vi "Insert Channel Create Params.vi"(8 "error in":errorcluster, 11 "TDMS in":refnum<class "TDMS.lvclass">) -> (0 "error out":errorcluster, 3 "TDMS out":refnum<class "TDMS.lvclass">)   [LabVIEW 2019, in "TDMS.lvlib" / "TDMS.lvclass"]
uses:
  TDMS.lvclass
  TDMS.lvclass/TDMS.ctl
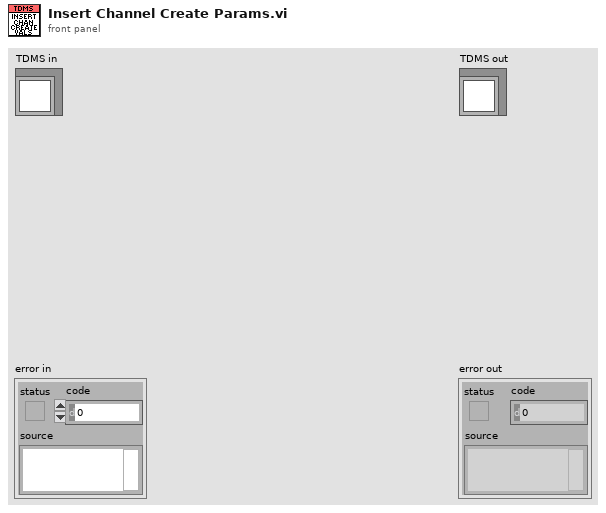
[diagram p1: front panel]
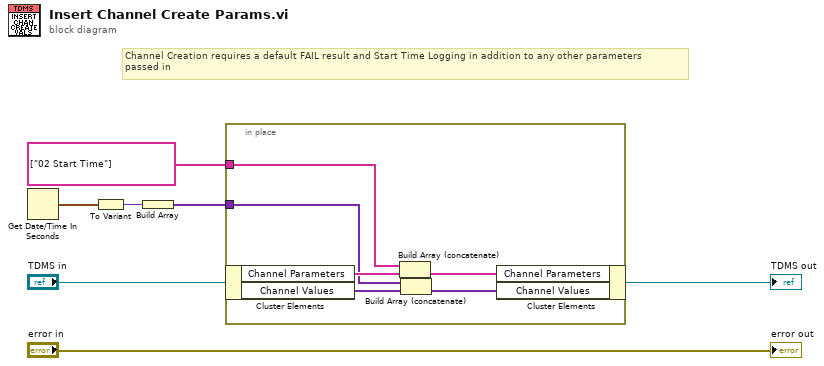
[diagram p0: block diagram]
diagram:
  # "Channel Creation requires a default FAIL result and Start Time Logging in addition to any other parameters \npassed in"
  n1 = Get Date/Time In Seconds() -> (seconds since 1Jan1904=w7:timestamp)
  n2 = To Variant(anything=w7) -> (Variant=w4:variant)
  n3 = Build Array(w4) -> (w3:variant[])
  n4 = in-place {
    in-place-border: string[] ["02 Start Time"] -> [w11]
    in-place-border: w3 -> [w8]
    n5 = in-place-cluster #1("TDMS in") -> ("Channel Parameters"=w13:string[], "Channel Values"=w10:variant[])
    n6 = Build Array (concatenate)(w11, w13) -> (w12:string[])
    n7 = Build Array (concatenate)(w8, w10) -> (w9:variant[])
    n8 = in-place-cluster #1("Channel Parameters"=w12, "Channel Values"=w9) -> (→"TDMS out":refnum<class "TDMS.lvclass">)
  }
  "error out" <- "error in"
